vi "OFDM TX_syh.vi"() -> ()   [LabVIEW 2013]
uses:
  <vilib>/addons/Modulation/Analog/controls/Complex Data Waveform.ctl
  <vilib>/Analysis/2dsp.llb/Inverse Complex FFT.vi
  <vilib>/addons/Modulation/Digital/General/MT Generate Bits (Galois, PN Order).vi
  <vilib>/addons/Modulation/Digital/General/MT Map Bits to QAM Symbols.vi
  <vilib>/addons/Modulation/niDMT.lvlib
  <vilib>/Analysis/NI_AALPro.lvlib
  <vilib>/addons/Modulation/niAMT.lvlib
panel:
  in  "desired sample rate (Hz)":dbl=1.0 format="%.2f"
  out "Complex baseband":cluster{"t0":dbl, "dt":dbl, "Y":dbl[]}[](graph)
  in  "stop":bool
  out "error out":errorcluster
  in  "Queue size":i32
  out "output bit stream":i8[](array[numeric])
  out "Outgoing Constellation":cdb[](graph)
  in  "Number of Bits":i32=128
  in  "error in (no error)":errorcluster
  # "OFDM Transmitter"
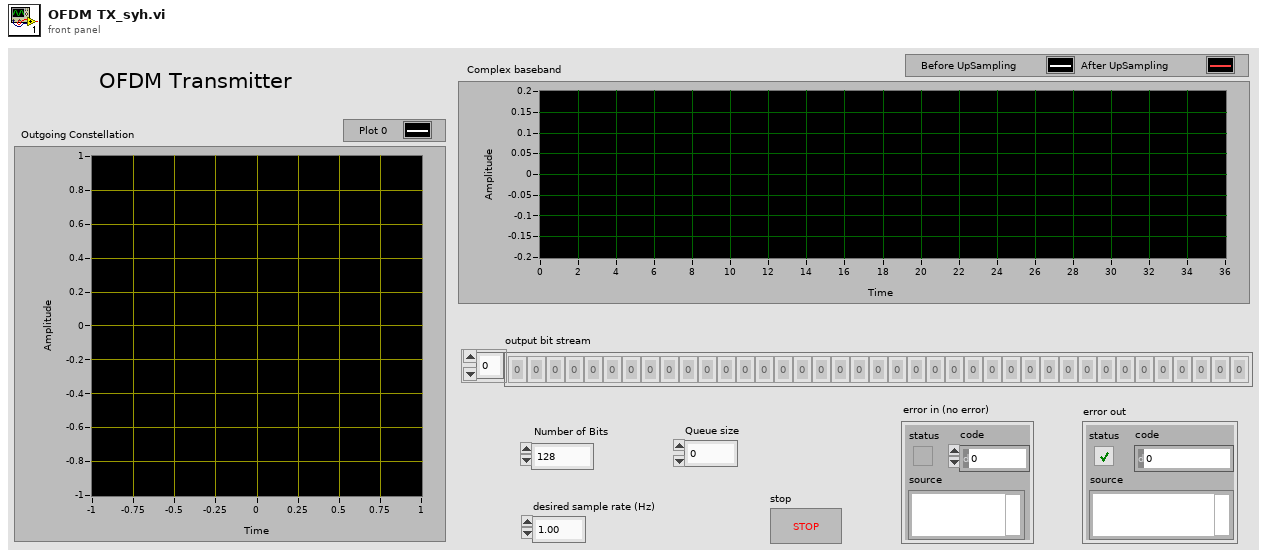
[diagram p1: front panel]
types:
  T1 = cluster{"IQ Data":cdb[], "Original Bitstream":i8[]}
  T2 = typedef "niAMT.lvlib/Complex Data Waveform.ctl" = cluster{"t0":dbl, "dt":dbl, "Y":cdb[]}
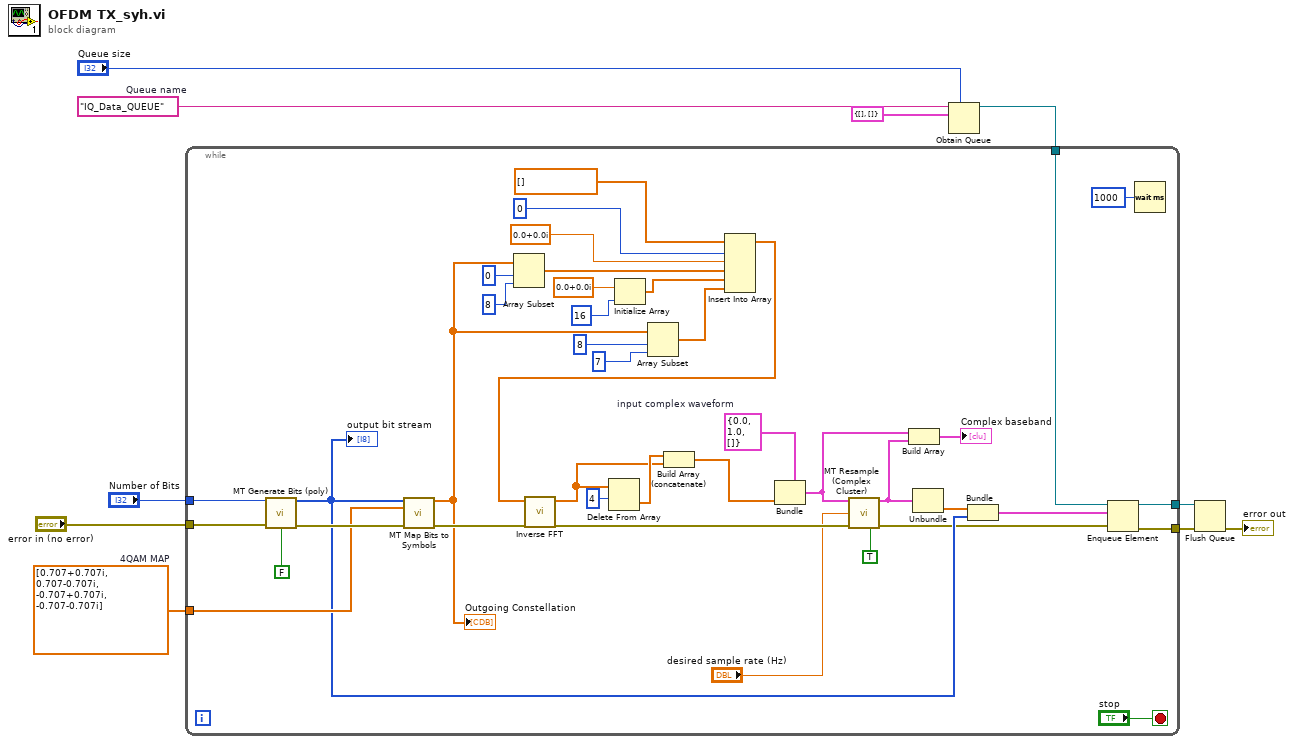
[diagram p0: block diagram]
diagram:
  w5 = cdb[] [0.707+0.707i, 0.707-0.707i, -0.707+0.707i, -0.707-0.707i]  # 4QAM MAP
  w8 = "IQ_Data_QUEUE"  # Queue name
  n1 = Obtain Queue(max queue size (-1, unlimited)="Queue size", name (unnamed)=w8, element data type=T1 {"IQ Data"=[], "Original Bitstream"=[]}) -> (queue out=w2:refnum<queue>)  [unwired: 2 in, 2 out]
  n2 = while {
    tunnel: "error in (no error)" -> [w48]
    tunnel: "Number of Bits" -> [w47]
    tunnel: w5 -> [w45]
    tunnel: [w37] -> w3
    tunnel: w2 -> [w36]
    tunnel: [w35] -> w1
    stop <- "stop" stop-if-true
    w29 = T2 {"t0"=0.0, "dt"=1.0, "Y"=[]}  # input complex waveform
    n3 = call-poly <vilib>:"MT Generate Bits (poly).vi"("total bits (128)"=w47, "error in (no error)"=w48, "reset? (T)"=FALSE) -> ("output bit stream"=w40:i8[], "error out"=w46:errorcluster)  [unwired: 10 in, 1 out]
    "output bit stream" <- w40
    n4 = call-poly <vilib>:"MT Map Bits to Symbols.vi"("input bit stream"=w40, "symbol map"=w45, "error in (no error)"=w46) -> ("symbols"=w19:cdb[], "error out"=w42:errorcluster)  [unwired: 11 in]
    "Outgoing Constellation" <- w19
    n5 = Array Subset(array=w19, index=0, length=8) -> (w23:cdb[])
    n6 = Initialize Array(cdb 0.0+0.0i ("element"), 16 ("dimension size")) -> (w20:cdb[])
    n7 = Array Subset(array=w19, index=8, length=7) -> (w12:cdb[])
    n8 = Insert Into Array(array=cdb[] [], index=0, new element #1=cdb 0.0+0.0i ("element"), new element #2=w23, new element #3=w20, new element #4=w12) -> (w15:cdb[])
    n9 = call-poly <vilib>:"Inverse FFT.vi"("FFT {X}"=w15) -> ("X"=w26:cdb[])  [unwired: 9 in, 1 out]
    n10 = Delete From Array(array=w26, length=4) -> (deleted portion=w27:cdb[])  [unwired: 1 in, 1 out]
    n11 = Build Array (concatenate)(w27, w26) -> (w11:cdb[])
    n12 = Bundle(cluster=w29, "Y"=w11) -> (w32:T2)  [unwired: 2 in]
    n13 = call <vilib>:"MT Resample (Complex Cluster).vi"("input complex waveform"=w32, "desired sample rate (Hz)"="desired sample rate (Hz)", "error in (no error)"=w42, "flush buffers? (F)"=TRUE) -> ("output complex waveform"=w33:T2, "error out"=w38:errorcluster)  [unwired: 10 in]
    n14 = Build Array(w32, w33) -> (→"Complex baseband":T2[])
    n15 = Unbundle(w33) -> ("Y"=w41:cdb[])  [unwired: 2 out]
    n16 = Bundle("Y"=w41, "output bit stream"=w40) -> (w39:cluster{"Y":cdb[], "output bit stream":i8[]})  [unwired: 1 in]
    n17 = Enqueue Element(queue=w36, element=w39, error in (no error)=w38) -> (queue out=w35:refnum<queue>, error out=w37:errorcluster)  [unwired: 1 in, 1 out]
    n18 = Wait (ms)(milliseconds to wait=u32 1000) -> ()  [unwired: 1 out]
  }
  n19 = Flush Queue(queue=w1, error in (no error)=w3) -> (error out=→"error out":errorcluster)  [unwired: 2 out]
